vi "emi_Read Keys.vi"(0 "Ini Path(..app../config.ini)":path=path "", 1 "Section":string, 5 "Key Names":string[](array[string]), 7 "Types/Defaults":variant[](array[variant]), 11 "error in (no error)":errorcluster) -> (6 "file created?":bool, 8 "Values":variant[](array[variant]), 15 "error out":errorcluster)   [LabVIEW 2011]
doc: "Write numerous keys into ini file. Creates and openes ini file id \\\\s needed"
uses:
  App/emi_Application Folder.vi
  <vilib>/Utility/libraryn.llb/Check if File or Folder Exists.vi
  <vilib>/Utility/config.llb/NI_LVConfig.lvlib
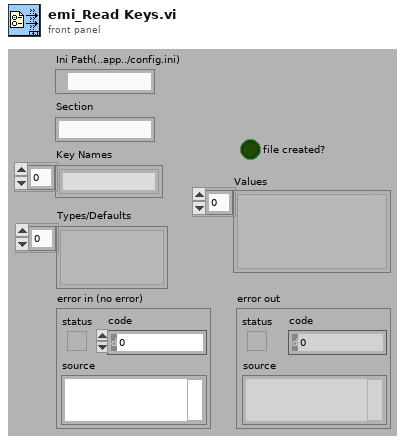
[diagram p1: front panel]
types:
  T1 = typedef "NI_LVConfig.lvlib/Config Data RefNum.ctl" = refnum<k1>
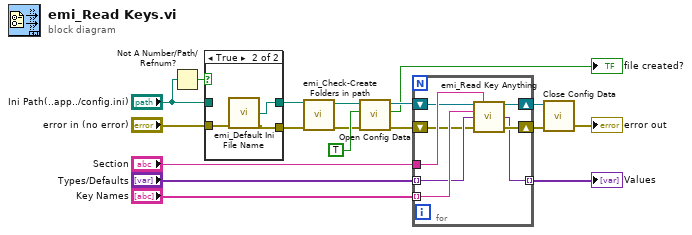
[diagram p0: block diagram]
diagram:
  n1 = Not A Number/Path/Refnum?(number/path/refnum="Ini Path(..app../config.ini)") -> (NaN/Path/Refnum?=w8:bool)
  n2 = case shown="True" w8 {
    tunnel: [w20 w22] -> w5
    tunnel: "Ini Path(..app../config.ini)" -> [w20 _]
    tunnel: "error in (no error)" -> [w19 w23]
    tunnel: [w19 w21] -> w6
    frame False {
    }
    frame True {
      n3 = call "emi_Default Ini File Name.vi"("error in (no error)"=w23) -> ("Path"=w22:path, "error out"=w21:errorcluster)  [unwired: 13 in]
    }
  }
  n4 = call "emi_Check-Create Folders in path.vi"("Path including file"=w5, "error in (no error)"=w6) -> ("Path out"=w3:path, "error out"=w4:errorcluster)  [unwired: 11 in, 1 out]
  n5 = call <vilib>:"Open Config Data.vi"("error in (no error)"=w4, "create file if necessary (T)"=TRUE, "configuration file path"=w3) -> ("error out"=w13:errorcluster, "file created?"=→"file created?":bool, "refnum"=w14:T1)  [unwired: 6 in]
  n6 = for {
    tunnel: "Section" -> [w31]
    tunnel: "Types/Defaults" -> [w28] mode=indexing
    tunnel: "Key Names" -> [w29] mode=indexing
    shift-right: [w26] -> w11
    shift-left: w13 -> [w27]
    shift-right: [w25] -> w12
    shift-left: w14 -> [w30]
    tunnel: [w24] -> w2 mode=indexing
    n7 = call "emi_Read Key Anything.vi"("Ini file refnum"=w30, "Section(Default)"=w31, "Name"=w29, "Anything"=w28, "error in (no error)"=w27) -> ("Ini file refnum out"=w25:T1, "Anything Out"=w24:variant, "error out"=w26:errorcluster)  [unwired: 7 in, 1 out]
  }
  "Values" <- w2
  n8 = call <vilib>:"Close Config Data.vi"("error in (no error)"=w11, "refnum"=w12) -> ("error out"=→"error out":errorcluster)  [unwired: 8 in, 1 out]
